vi "TEST_Eurotherm_1ch.vi"() -> ()   [LabVIEW 2017]
uses:
  Eurotherm_Setpoint Control.ctl
  Address.ctl
  Eurotherm_2023_Module.ctl
panel:
  out "Eurotherm":T1
  in  "SP":bool=TRUE
  in  "Address":T2
  in  "WRITE PID":bool
  in  "PID":cluster{"kP":dbl, "kI":dbl, "kD":dbl}={"kP"=50.0, "kI"=120.0, "kD"=600.0}
  in  "Write":T3 {"Rate (C/min)" min=0.0 max=99.9 step=0.1 format="%.1f"; "Setpoint (C)" min=-100.0 max=100.0 step=0.1 format="%.1f"}
  in  "READ":bool
  in  "WRITE SP":bool
  in  "stop":bool
  out "error in (no error)":errorcluster
  in  "VISA resource name":refnum<visa-resource-name>="COM1"
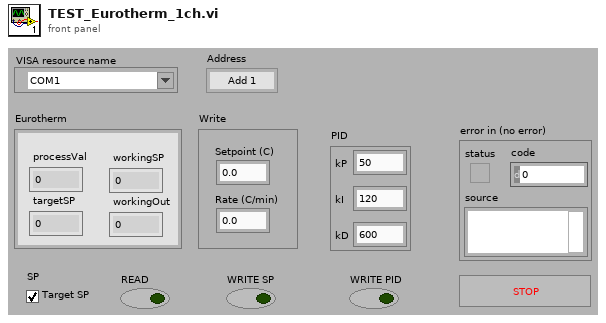
[diagram p1: front panel]
types:
  T1 = cluster{"processVal":dbl, "targetSP":dbl, "workingSP":dbl, "workingOut":dbl}
  T2 = typedef "Address.ctl" = enum16{"Add 1", "Add 2", "Add 3", "Add 4", "Add 5", "Add 6", "Add 10", "Add 11", "Add 12", "Add 13"}
  T3 = typedef "Eurotherm_Setpoint Control.ctl" = cluster{"Setpoint (C)":dbl, "Rate (C/min)":dbl}
  T4 = typedef "Eurotherm_2023_Module.ctl" = enum16{"Initialize", "Write setpoint", "Read data", "Write ramp rate", "Set constante proporcional", "Set constante integral", "Set constante diferencial", "Set ouput limit LOW", "Set ouput limit HIGH", "Shutdown"}
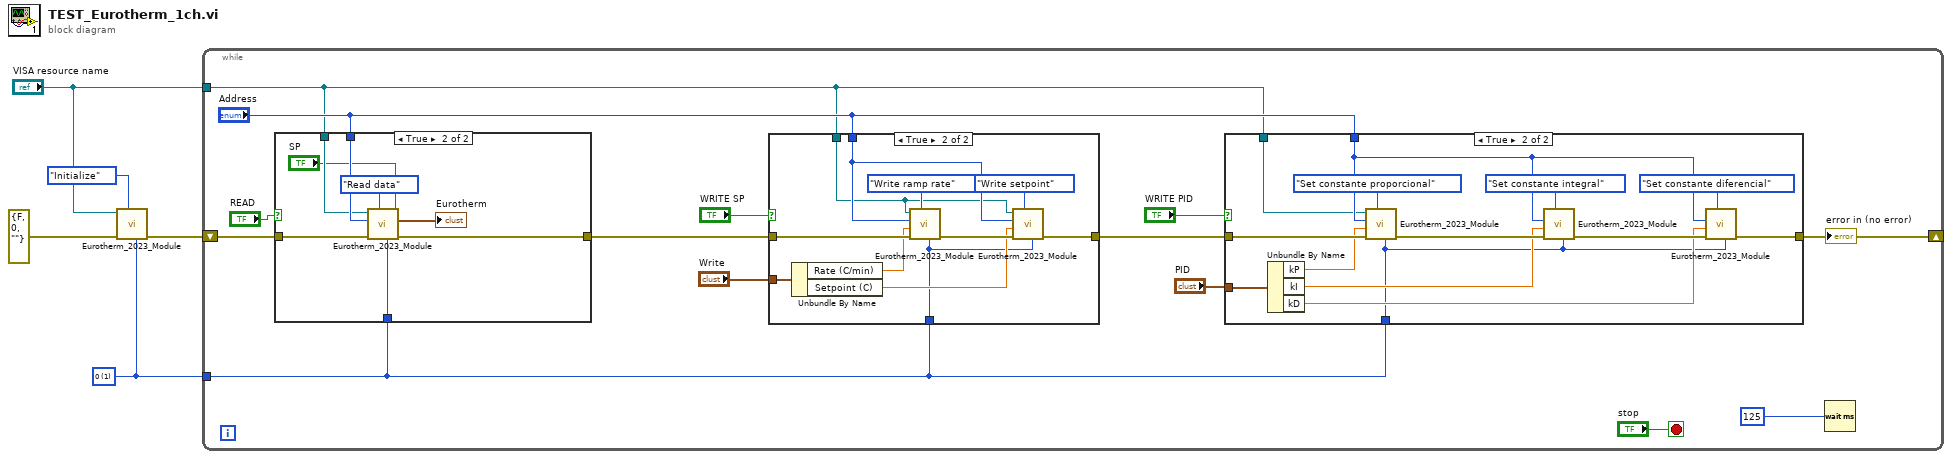
[diagram p0: block diagram]
diagram:
  w2 = u16 1 items=["0"=1, "1"=10, "2"=100] ("Decimales")
  n1 = call "Eurotherm_2023_Module.vi"("Decimales"=w2, "Command"=Eurotherm_2023_Module."Initialize", "error in (no error)"=errorcluster {"status"=FALSE, "code"=0, "source"=""}, "VISA resource name"="VISA resource name") -> ("error out"=w3:errorcluster)  [unwired: 6 in, 1 out]
  n2 = while {
    shift-right: [w10] -> _
    shift-left: w3 -> [w18]
    tunnel: w2 -> [w9]
    tunnel: "VISA resource name" -> [w6]
    stop <- "stop" stop-if-true
    n3 = case shown="True" "READ" {
      tunnel: w18 -> [w47 w55]
      tunnel: [w47 w54] -> w17
      tunnel: w9 -> [_ w52]
      tunnel: "Address" -> [_ w51]
      tunnel: w6 -> [_ w50]
      frame False {
      }
      frame True {
        n4 = call "Eurotherm_2023_Module.vi"("SP"="SP", "Decimales"=w52, "Command"=Eurotherm_2023_Module."Read data", "error in (no error)"=w55, "Address"=w51, "VISA resource name"=w50) -> ("error out"=w54:errorcluster, "Eurotherm"=→"Eurotherm":T1)  [unwired: 4 in]
      }
    }
    n5 = case shown="True" "WRITE SP" {
      tunnel: w17 -> [w35 w46]
      tunnel: [w35 w44] -> w11
      tunnel: "Write" -> [_ w41]
      tunnel: w9 -> [_ w38]
      tunnel: "Address" -> [_ w37]
      tunnel: w6 -> [_ w36]
      frame False {
      }
      frame True {
        n6 = Unbundle By Name(w41) -> ("Rate (C/min)"=w40:dbl, "Setpoint (C)"=w39:dbl)
        n7 = call "Eurotherm_2023_Module.vi"("Decimales"=w38, "Command"=Eurotherm_2023_Module."Write ramp rate", "error in (no error)"=w46, "Value"=w40, "Address"=w37, "VISA resource name"=w36) -> ("error out"=w45:errorcluster)  [unwired: 4 in, 1 out]
        n8 = call "Eurotherm_2023_Module.vi"("Decimales"=w38, "Command"=Eurotherm_2023_Module."Write setpoint", "error in (no error)"=w45, "Value"=w39, "Address"=w37, "VISA resource name"=w36) -> ("error out"=w44:errorcluster)  [unwired: 4 in, 1 out]
      }
    }
    n9 = case shown="True" "WRITE PID" {
      tunnel: w11 -> [w20 w34]
      tunnel: [w20 w25] -> w10
      tunnel: "PID" -> [_ w30]
      tunnel: w9 -> [_ w23]
      tunnel: "Address" -> [_ w22]
      tunnel: w6 -> [_ w21]
      frame False {
      }
      frame True {
        n10 = Unbundle By Name(w30) -> ("kP"=w29:dbl, "kI"=w28:dbl, "kD"=w24:dbl)
        n11 = call "Eurotherm_2023_Module.vi"("Decimales"=w23, "Command"=Eurotherm_2023_Module."Set constante proporcional", "error in (no error)"=w34, "Value"=w29, "Address"=w22, "VISA resource name"=w21) -> ("error out"=w33:errorcluster)  [unwired: 4 in, 1 out]
        n12 = call "Eurotherm_2023_Module.vi"("Decimales"=w23, "Command"=Eurotherm_2023_Module."Set constante integral", "error in (no error)"=w33, "Value"=w28, "Address"=w22) -> ("error out"=w26:errorcluster)  [unwired: 5 in, 1 out]
        n13 = call "Eurotherm_2023_Module.vi"("Decimales"=w23, "Command"=Eurotherm_2023_Module."Set constante diferencial", "error in (no error)"=w26, "Value"=w24, "Address"=w22) -> ("error out"=w25:errorcluster)  [unwired: 5 in, 1 out]
      }
    }
    "error in (no error)" <- w10
    n14 = Wait (ms)(milliseconds to wait=u32 125) -> ()  [unwired: 1 out]
  }
